vi "ReScan.vi"(8 "error in (no error)":errorcluster, 10 "s":bool, 11 "Data In":T2) -> (0 "error out":errorcluster, 1 "States":T1, 3 "Data Out":T2)   [LabVIEW 2014]
uses:
  controls/ReadScan1States.ctl
  controls/State.ctl
  controls/Data1.ctl
panel:
  in  "number":u32
  # "日      期"
  # "機       種"
  # "機       號"
  # "商品條碼"
  # "OK"
  # "台"
  # "NG"
  # "台"
  # "總計"
  # "台"
  # "日      期"
  # "機       種"
  # "機       號"
  # "商品條碼"
  # "OK"
  # "台"
  # "NG"
  # "台"
  # "總計"
  # "台"
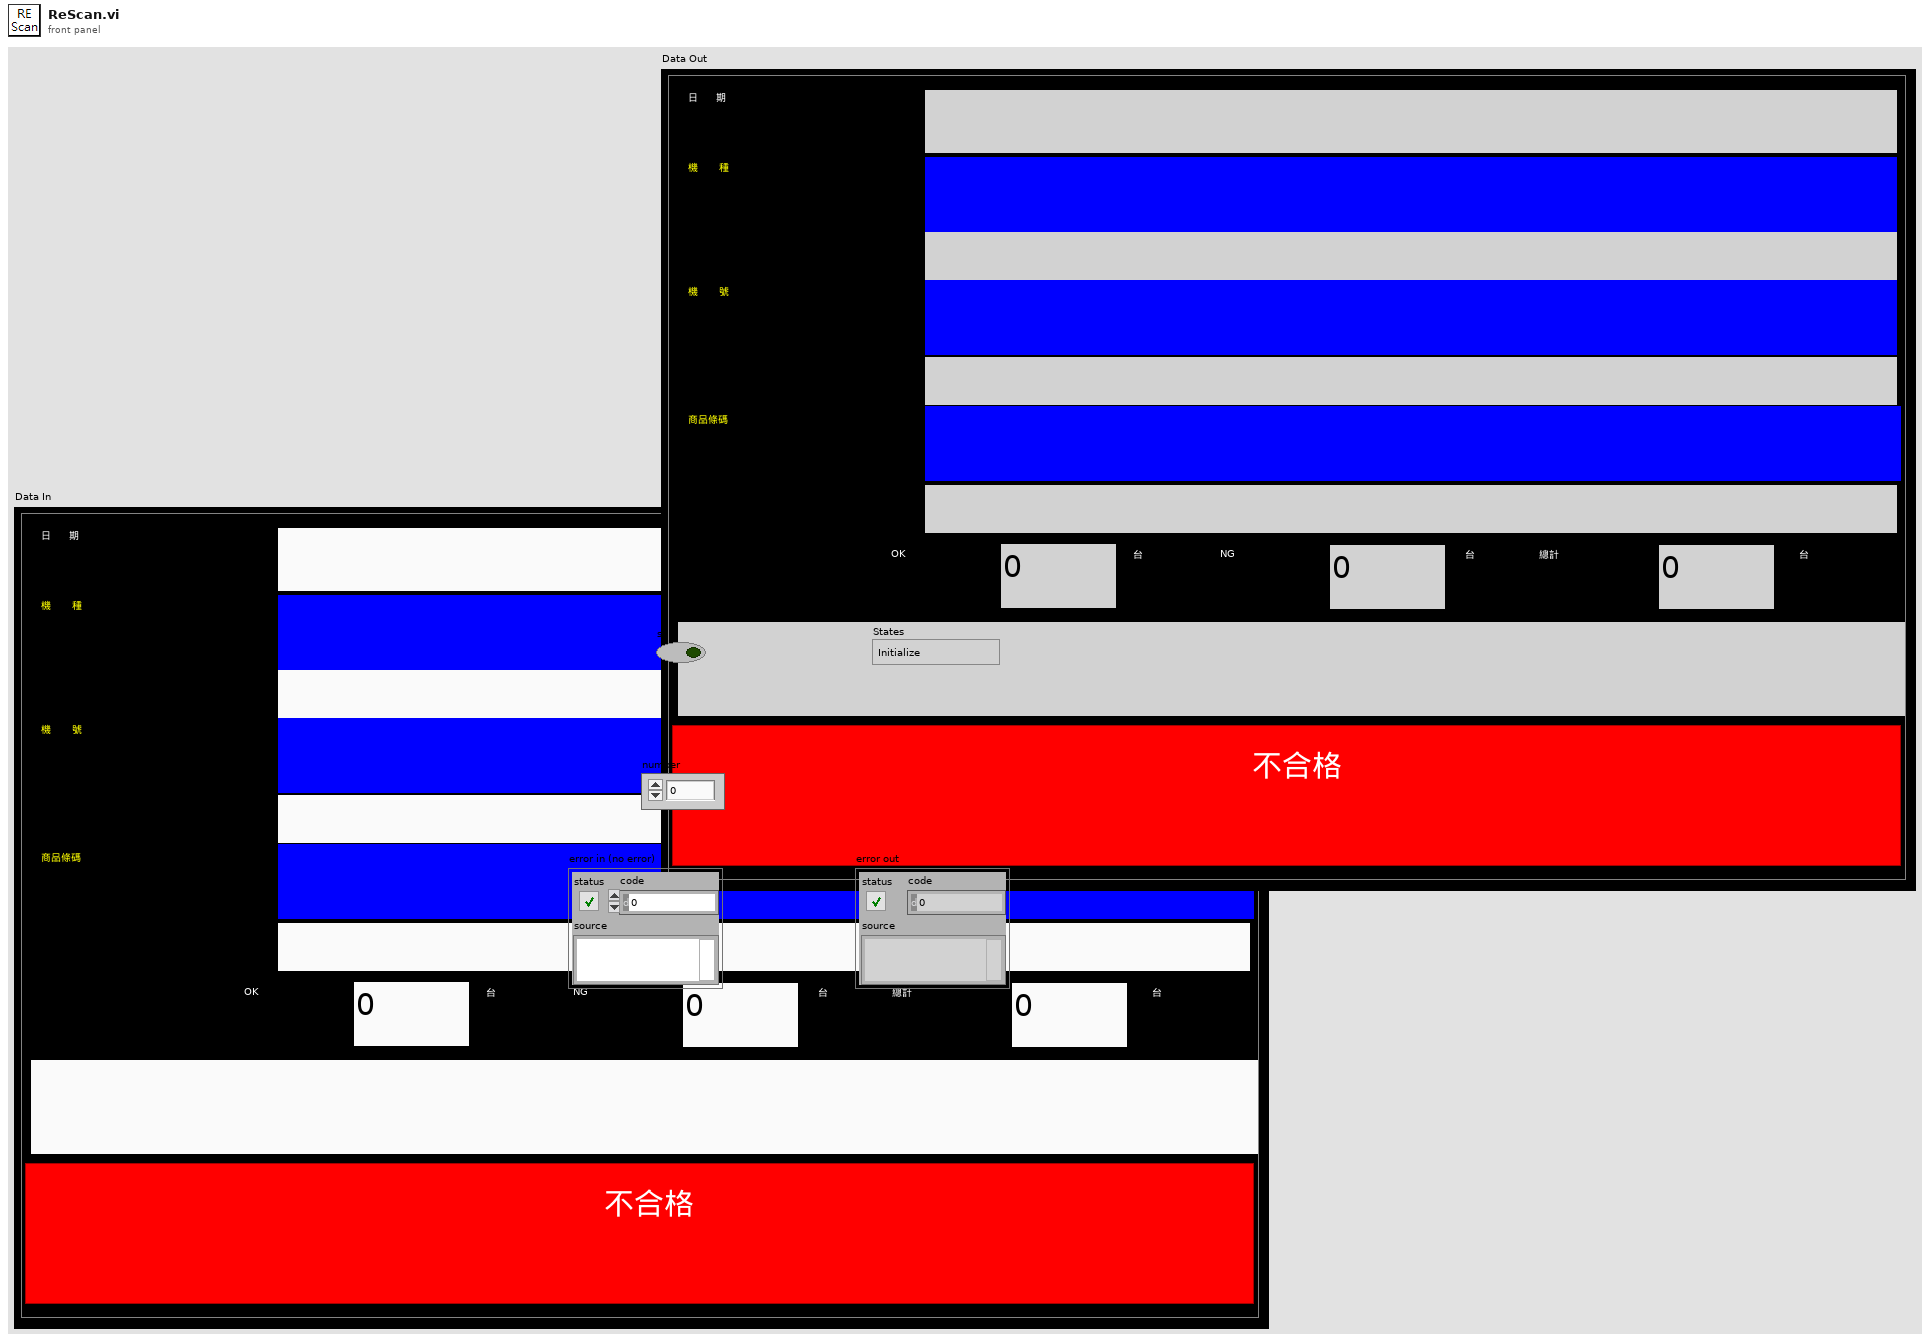
[diagram p1: front panel]
types:
  T1 = typedef "State.ctl" = enum16{"Initialize", "Wait for Scan", "State 1", "State 2", "NG", "NG1", "OK", "OKNG", "OKNG1", "Exit"}
  T2 = typedef "Data1.ctl" = cluster{"Date":string, "BarCode1":string, "BarCode2":string, "BarCode3":string, "Message":string, "OK Count":u16, "NG Count":u16, "Total Count":u16, "ModelData":string[][], "OK&NG":bool, "COM1":refnum<visa-resource-name>, "COM2":refnum<visa-resource-name>, "IO":i32, "Time":u32, "TCP":refnum<k5>, "TCP 2":refnum<k5>, "COM1 2":refnum<visa-resource-name>, "CheckPars":string, "BarCode1_1":string, "BarCode2_1":string, "BarCode3_1":string}
  T3 = typedef "ReadScan1States.ctl" = enum16{"Initialize", "Init2", "Step1", "Step2", "Step3", "Step4", "One", "Two", "Three", "Four", "Five", "End", "Stop"}
  T4 = typedef "Data1.ctl" = cluster{"Date":string, "BarCode1":string, "BarCode2":string, "BarCode3":string, "Message":string, "OK Count":u16, "NG Count":u16, "Total Count":u16, "ModelData":string[][], "OK&NG":bool, "COM1":refnum<visa-resource-name>, "COM2":refnum<visa-resource-name>, "IO":i32, "Time":u32, "TCP":refnum<k5>, "TCP 2":refnum<k5>, "COM1 2":refnum<visa-resource-name>, "CheckNum":string, "BarCode1_1":string, "BarCode2_1":string, "BarCode3_1":string, "日期":string, "機種":string, "機號":string, "商品條碼1":string, "OK_1":string, "OK":string, "NG":string, "NG_1":string, "Total":string, "Total_1":string, "ClaerTime":u32, "Pjson":T5, "LotNo":string[], "CheckParsArray":string[], "BarCode4":string, "BarCode4_1":string, "商品條碼2":string, "BarCode5":string, "BarCode5_1":string, "商品條碼3":string, "ReScanNG":i32, "NGTimeCT":u32}
  T5 = typedef "Payjson.ctl" = cluster{"DEPT":string, "LINE":string, "STANO":string, "WORKNO":string, "PRODSN":string, "COMPNTID":string, "COMPNTLOT":string, "COMPNTSN":string, "USEDQTY":i16, "OPDATE":string, "OPUSER":string, "RECVDATE":string, "MMODU":string}[]
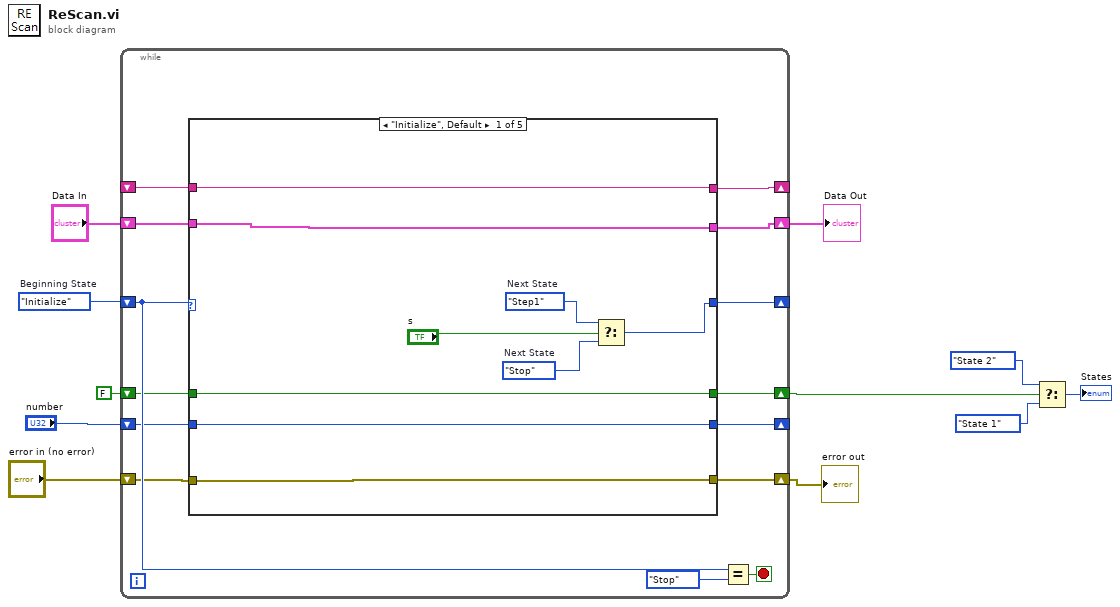
[diagram p0: block diagram]
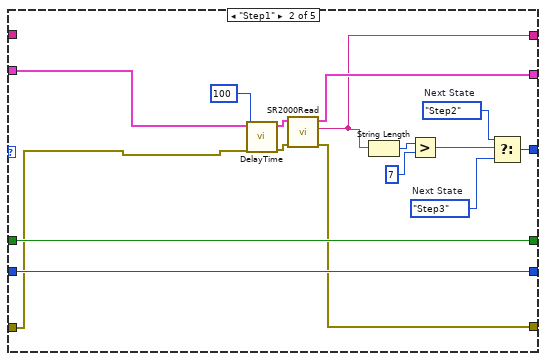
[diagram p2: hidden frame]
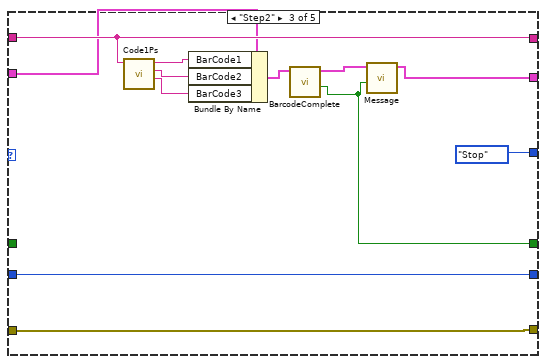
[diagram p3: hidden frame]
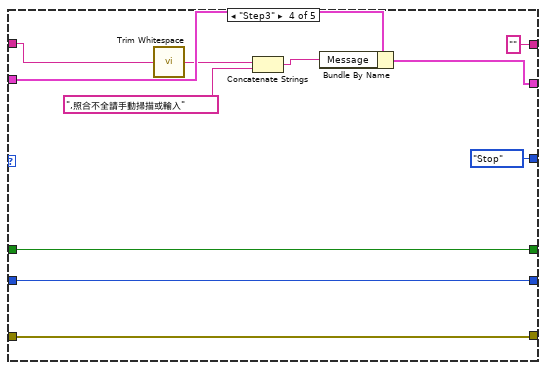
[diagram p4: hidden frame]
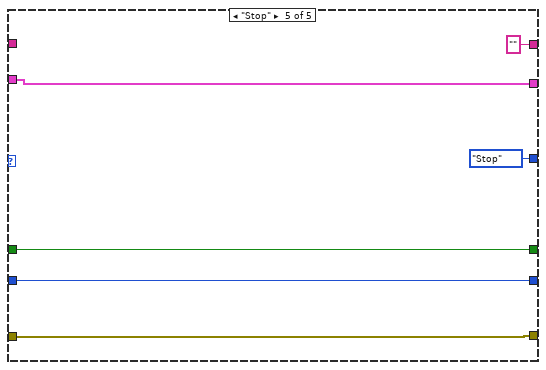
[diagram p5: hidden frame]
diagram:
  w11 = ReadScan1States."Initialize"  # Beginning State
  n1 = while {
    shift-right: [w22] -> _
    shift-left: w11 -> [w23]
    shift-right: [w17] -> w9
    shift-left: "Data In" -> [w20]
    shift-right: [w16] -> w7
    shift-left: "error in (no error)" -> [w21]
    shift-right: [w18] -> _
    shift-left: _ -> [w19]
    shift-right: [w15] -> w4
    shift-left: FALSE -> [w14]
    shift-right: [w12] -> _
    shift-left: "number" -> [w13]
    stop <- w25 stop-if-true
    n2 = case shown="\"Initialize\", Default" w23 {
      tunnel: [w32 w45 ReadScan1States."Stop" ("Next State") ReadScan1States."Stop" ("Next State") ReadScan1States."Stop" ("Next State")] -> w22
      tunnel: w21 -> [w26 w35 w60 w72 w76]
      tunnel: w20 -> [w27 w36 w61 w69 w77]
      tunnel: w19 -> [w29 _ w62 w64 _]
      tunnel: [w29 w43 w62 "" ("BarCodeRead") ""] -> w18
      tunnel: [w27 w47 w52 w68 w77] -> w17
      tunnel: [w26 w48 w60 w72 w76] -> w16
      tunnel: [w31 w50 w51 w71 w75] -> w15
      tunnel: w14 -> [w31 w50 _ w71 w75]
      tunnel: w13 -> [w30 w49 w58 w70 w74]
      tunnel: [w30 w49 w58 w70 w74] -> w12
      frame "Initialize", Default {
        w34 = ReadScan1States."Step1"  # Next State
        w33 = ReadScan1States."Stop"  # Next State
        n3 = Select(t=w34, s="s", f=w33) -> (s? t:f=w32:T3)
      }
      frame "Step1" {
        w44 = ReadScan1States."Step3"  # Next State
        w46 = ReadScan1States."Step2"  # Next State
        n4 = call "DelayTime.vi"("error in (no error)"=w35, "Time"=u32 100, "Data In"=w36) -> ("error out"=w38:errorcluster, "Data Out"=w39:T4)  [unwired: 7 in]
        n5 = call "SR2000Read.vi"("error in (no error)"=w38, "Data In"=w39) -> ("error out"=w48:errorcluster, "BarCodeRead"=w43:string, "Data Out"=w47:T2)  [unwired: 7 in]
        n6 = String Length(string=w43) -> (length=w42:i32)
        n7 = Greater?(x=w42, y=7) -> (0:w40:bool)
        n8 = Select(t=w46, s=w40, f=w44) -> (s? t:f=w45:T3)
      }
      frame "Step2" {
        n9 = call "Code1Ps.vi"("Code1 In"=w62) -> ("紙箱號碼"=w55:string, "機種代號"=w56:string, "機種名"=w57:string)  [unwired: 8 in]
        n10 = Bundle By Name(cluster=w61, "BarCode1"=w57, "BarCode2"=w56, "BarCode3"=w55) -> (w54:T2)
        n11 = call "BarcodeComplete.vi"("Data In"=w54) -> ("Complete"=w51:bool, "Data Out"=w53:T4)  [unwired: 9 in]
        n12 = call "Message.vi"("TorF"=w51, "Data In"=w53) -> ("Data Out"=w52:T2)  [unwired: 9 in]
      }
      frame "Step3" {
        n13 = call <vilib>:"Trim Whitespace.vi"("string"=w64) -> ("trimmed string"=w63:string)  [unwired: 1 in]
        n14 = Concatenate Strings(w63, ",照合不全請手動掃描或輸入" ("string")) -> (w66:string)
        n15 = Bundle By Name(cluster=w69, "Message"=w66) -> (w68:T2)
      }
      frame "Stop" {
      }
    }
    n16 = Equal?(x=w23, y=ReadScan1States."Stop" ("States")) -> (x = y?=w25:bool)
  }
  "Data Out" <- w9
  "error out" <- w7
  n17 = Select(t=State."State 2" ("States"), s=w4, f=State."State 1" ("States")) -> (s? t:f=→"States":T1)
